vi "UI_update_Zone_indicator_params_(univ).vi"(8 "error in (no error)":errorcluster, 10 "Geometry":T1 {"Cage type" items=["Round", "Square", "Donut-maze", "T-maze", "Sociability maze", ""]}, 11 "Zone indicator ref. in":refnum<vi>) -> (0 "error out":errorcluster, 3 "Zone indicator ref. out":refnum<vi>)   [LabVIEW 2018, in "Tracker.lvlib"]
uses:
  Tracker.lvlib
  Controls/CTL_Segmented_plot_parameters_2.ctl
  Libraries/Cage Diagram/Typedefs/CTL_Cage_type.ctl
  Controls/CTL_Cage_all_segmentation_params_set.ctl
  Controls/CTL_Segmented_plot_parameters_2_(round_d1).ctl
  Common_Resources.lvlib
  Libraries/Cage Diagram/Cage Diagram.lvlib
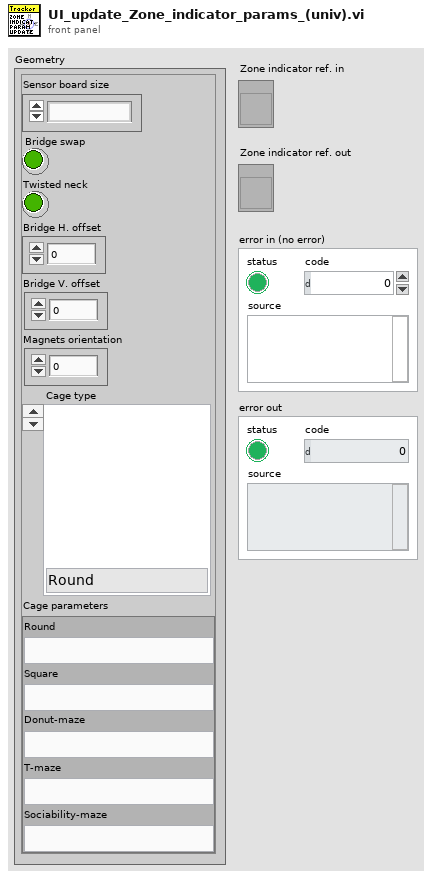
[diagram p1: front panel]
types:
  T1 = typedef "Common_Resources.lvlib/CTL_Segmented_plot_parameters_2.ctl" = cluster{"Sensor board size":enum16{"", "Large"}, "Bridge swap":bool, "Twisted neck":bool, "Bridge H. offset":sgl, "Bridge V. offset":sgl, "Magnets orientation":sgl, "Cage type":T2, "Cage parameters":T3}
  T2 = typedef "Cage Diagram.lvlib/CTL_Cage_type.ctl" = u16
  T3 = typedef "Common_Resources.lvlib/CTL_Cage_all_segmentation_params_set.ctl" = cluster{"Round":variant, "Square":variant, "Donut-maze":variant, "T-maze":variant, "Sociability-maze":variant}
  T4 = typedef "Common_Resources.lvlib/CTL_Segmented_plot_parameters_2_(round_d1).ctl" = cluster{"Cage diameter, mm":u16, "Starting angle BORDER":i16, "Starting angle MIDFIELD":i16, "Radius, mm MIDFIELD":u16, "Radius, mm CENTER":u16, "N segments BORDER":u8, "N segments MIDFIELD":u8, "R-gap, mm":sgl}
  T5 = enum8{"Enabled", "Disabled", "Disabled and Grayed Out"}
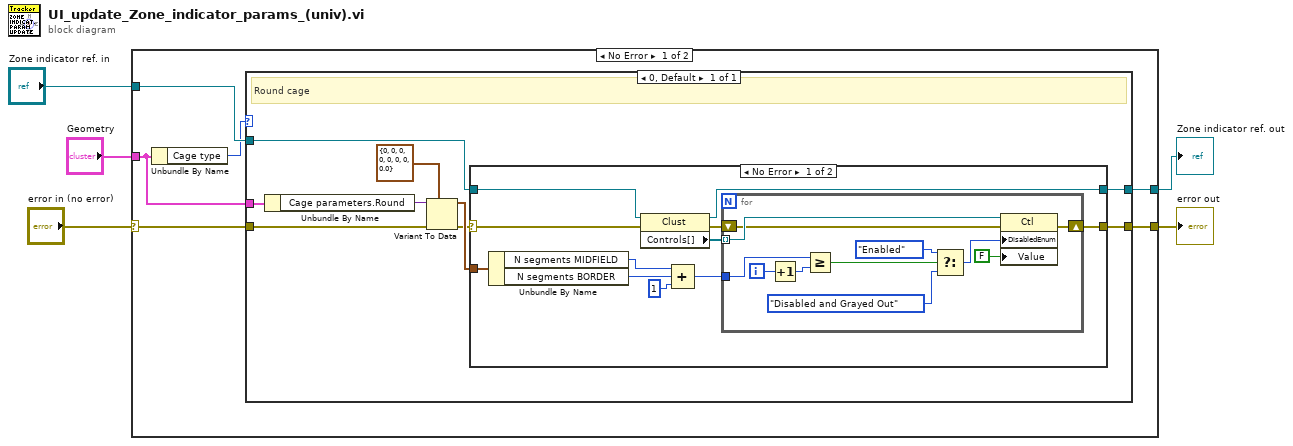
[diagram p0: block diagram]
diagram:
  n1 = case shown="No Error" "error in (no error)" {
    selector: "error in (no error)" -> [w8 w46]
    tunnel: [w11 w46] -> w5
    tunnel: "Zone indicator ref. in" -> [w10 w45]
    tunnel: [w9 w45] -> w3
    tunnel: "Geometry" -> [w6 _]
    frame No Error {
      n2 = Unbundle By Name(w6) -> ("Cage type"=w7:T2)
      n3 = case shown="0, Default" w7 {
        tunnel: [w20] -> w11
        tunnel: w10 -> [w19]
        tunnel: [w18] -> w9
        tunnel: w8 -> [w15]
        tunnel: w6 -> [w17]
        frame 0, Default {
          # "Round cage"
          n4 = Unbundle By Name(w17) -> ("Cage parameters.Round"=w16:variant)
          n5 = Variant To Data(error in=w15, type=T4 {"Cage diameter, mm"=0, "Starting angle BORDER"=0, "Starting angle MIDFIELD"=0, "Radius, mm MIDFIELD"=0, "Radius, mm CENTER"=0, "N segments BORDER"=0, "N segments MIDFIELD"=0, "R-gap, mm"=0.0} ("Geometry params in"), Variant=w16) -> (data=w13:T4, error out=w12:errorcluster)
          n6 = case shown="No Error" w12 {
            selector: w12 -> [w21 w44]
            tunnel: [w31 w44] -> w20
            tunnel: w19 -> [w24 w43]
            tunnel: [w23 w43] -> w18
            tunnel: w13 -> [w22 _]
            frame No Error {
              n7 = Unbundle By Name(w22) -> ("N segments MIDFIELD"=w27:u8, "N segments BORDER"=w28:u8)
              n8 = property class="Clust"(reference=w24, error in=w21) -> (reference out=w23:refnum<vi>, error out=w30:errorcluster, "Controls[]"=w25:refnum<vi>[])
              n9 = Compound Arithmetic op=ADD(w27, w28, u8 1 ("value")) -> (w29:u8)
              n10 = for {
                tunnel: w25 -> [w37] mode=indexing
                tunnel: w29 -> [w33]
                shift-right: [w35] -> w31
                shift-left: w30 -> [w36]
                i -> [w34]
                n11 = Increment(x=w34) -> (x+1=w39:i32)
                n12 = Greater Or Equal?(x=w33, y=w39) -> (x >= y?=w38:bool)
                n13 = Select(t=T5."Enabled" ("Disabled"), s=w38, f=T5."Disabled and Grayed Out") -> (s? t:f=w41:T5)
                n14 = property class="Ctl"(reference=w37, error in=w36, "DisabledEnum"=w41, "Value"=FALSE) -> (error out=w35:errorcluster)  [unwired: 1 out]
              }
            }
            frame Error {
            }
          }
        }
      }
    }
    frame Error {
    }
  }
  "error out" <- w5
  "Zone indicator ref. out" <- w3
